vi "FPGA_MPU_rev1.vi"() -> ()   [LabVIEW 2015]
uses:
  <vilib>/rvi/Emulation/niFpgaGetClockAttributes.vi
  <vilib>/rvi/Emulation/niFpgaSctlEmulationGetInTimedLoop.vi
  <vilib>/rvi/Emulation/niFpgaEmulationReportErrorSimple.vi
  <vilib>/rvi/eio/common/nirviEmuTemplateMethod_errors.vi
  <vilib>/rvi/Emulation/niFpgaCriticalErrorInLSC.vi
  <vilib>/eio/EIONode/EIONode.xnode
panel:
  in  "Count(Ticks)":u32=10
  in  "stop":bool
  in  "MOSI":bool
  in  "SCL":bool
  in  "CS":bool
  out "MISO":bool
  # "Entering a number (eg. 10) here will slow down the loop,\nYou may not want to use ax clock speed 40 MHz"
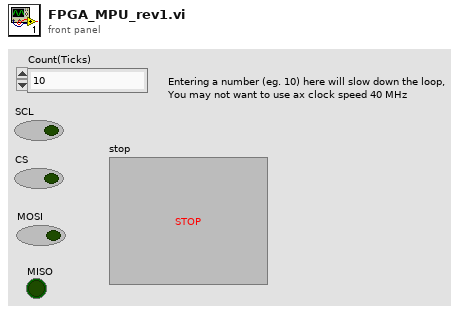
[diagram p1: front panel]
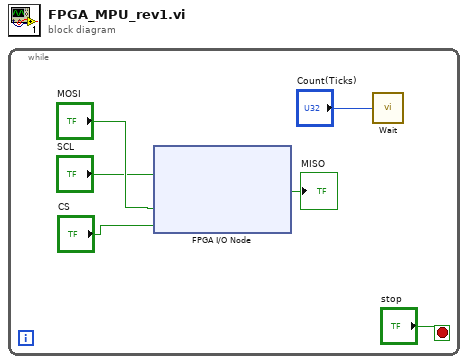
[diagram p0: block diagram]
diagram:
  n1 = while {
    stop <- "stop" stop-if-true
    n2 = xnode "FPGA I/O Node"("ConnectorB/DIO5"="SCL", "ConnectorB/DIO7"="MOSI", "ConnectorB/DIO1"="CS") -> ("ConnectorB/DIO6"=→"MISO":bool)  [unwired: 4 in, 4 out]
    n3 = call "Wait"("Count(Ticks)"="Count(Ticks)") -> ()  [unwired: 1 out]
  }
